vi "Real BC Test.vi"() -> ()   [LabVIEW 2016]
uses:
  Frames & Messages/TypeDefs/Message Config.ctl
  Frames & Messages/TypeDefs/Command Config.ctl
  Frames & Messages/TypeDefs/Message Control.ctl
  1553 SubComponent/TypeDefs/Parameter Table Data.ctl
  1553 SubComponent/TypeDefs/Scaling Information.ctl
  Bus Controller/TypeDefs/Bus Controller Configuration.ctl
  Frames & Messages/TypeDefs/Async Message Config.ctl
  Frames & Messages/TypeDefs/Async RT-RT Message Config.ctl
  1553 Board/1553 Board.lvclass/1553 Board.ctl
  Bus Controller/Bus Controller.lvclass
  D:/SVN/Products/BCI-1553/Software/Development/2016/RealTime/1553 SubComponent/1553 SubComponent.lvclass
  <vilib>/Utility/file.llb/Write Delimited Spreadsheet (string).vi
  1553 Component/1553 Component.lvclass
  Frames & Messages/Major Frame/Major Frame.lvclass
  1553 Board/1553 Board.lvclass
  Utilities/FPGA Interface/FPGA Interface.lvclass
  Frames & Messages/Async Message/Async Message.lvclass
  Frames & Messages/Message/Message.lvclass
  BCI-1553 API.lvlib
  1553 SubComponent/1553 SubComponent.lvclass
  Frames & Messages/Minor Frame/Minor Frame.lvclass
  Frames & Messages/Async RT-RT Message/Async RT-RT Message.lvclass
  D:/SVN/Products/BCI-1553/Software/Development/2016/RealTime/Frames & Messages/Async Message/Async Message.lvclass
panel:
  in  "Async Value":dbl format="%#_13g"
  in  "Async Param":string="Async Param"
  in  "Send Async":bool
  in  "Component ID (1-8)":u8=1
  in  "Update Param":bool
  in  "Scaled Data 2":dbl[](array[numeric])
  in  "Parameters 2":string[](array[string])
  out "Scaled Data":dbl[][](array[numeric])
  out "Parameters":string[][](array[string])
  in  "Holt Memory dump":path
  in  "Holt Memory to File":bool
  in  "Addresses to Read":u16 format="%0.0f"
  out "Data":u16[](array[numeric]) format="%04x"
  in  "Addr":u16 format="%04x"
  in  "Read":bool
  out "error out":errorcluster
  in  "stop":bool
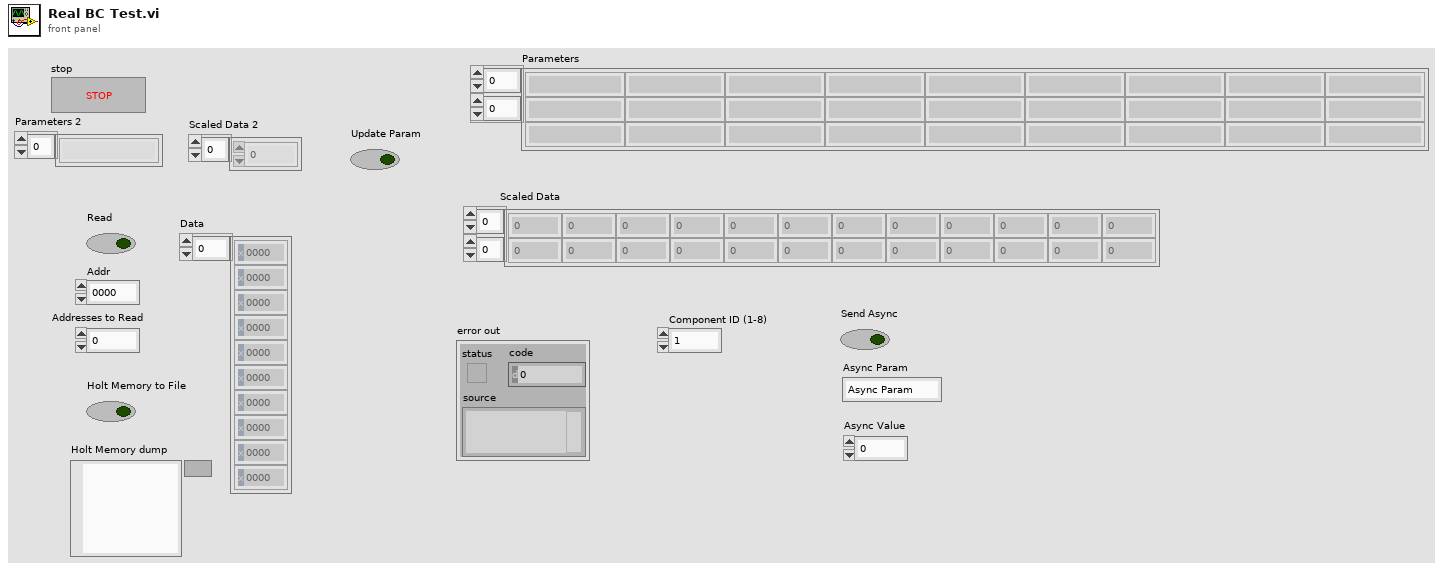
[diagram p1: front panel]
types:
  T1 = typedef "BCI-1553 API.lvlib/Async RT-RT Message Config.ctl" = cluster{"Tx Command Config":T2}
  T2 = typedef "BCI-1553 API.lvlib/Command Config.ctl" = cluster{"Command Type":enum16{"Transmit", "Receive"}, "Terminal Address (0-30)":u16, "SubAddress (1-30)":u16, "WC/MC (1-32)":u16, "Command Data":u16[]}
  T3 = typedef "BCI-1553 API.lvlib/1553 SubComponent.lvclass/Parameter Table Data.ctl" = cluster{"Parameter Name":string, "Base Word":u16, "Address":u16, "Value":u64, "Mask":u16[], "Scaling Info":T4}
  T4 = typedef "BCI-1553 API.lvlib/1553 SubComponent.lvclass/Scaling Information.ctl" = cluster{"Bit Offset":i32, "Bit Count":i32, "LSB Resolution":dbl, "2's Complement":bool, "Big Endian":bool, "Sign Bit":bool}
  T5 = typedef "BCI-1553 API.lvlib/Async Message Config.ctl" = cluster{"Group":i32, "High Priority":bool, "Time to Next Msg (100 us)":u16, "Command Config":T2, "Message Control":T6}
  T6 = typedef "BCI-1553 API.lvlib/Message Control.ctl" = cluster{"MC17 Time Sync":bool, "Error Mask":bool, "Service Request Mask":bool, "Busy Mask":bool, "SubSystem Flag Mask":bool, "Terminal Flag Mask":bool, "Reserved Mask":bool, "Retry":bool, "Bus A / !Bus B":bool, "Self-Test Loopback":bool, "Broadcast Mask":bool, "EoM Interrupt":bool, "Mode Code Format":bool, "Broadcast Format":bool, "RT-RT Format":bool}
  T7 = typedef "BCI-1553 API.lvlib/Message Config.ctl" = cluster{"Time to Next Msg (4 us)":u16, "Command Config":T2, "Message Control":T6}
  T8 = typedef "BCI-1553 API.lvlib/Bus Controller.lvclass/Bus Controller Configuration.ctl" = cluster{"BC Timeout":u16, "BC Retry":bool, "BC Second Retry":bool, "BC Retry Alt Bus":bool, "BC Second Retry Alt Bus":bool, "BC Retry on Status Bit":bool, "Msg Error No Data Valid":bool, "Busy Status No Data Valid":bool, "Msg Gap Timer":bool, "Watchdog Timer":bool, "Time Tag Sync":bool, "Even Time Tag Sync":bool, "Gap Check":bool, "Broadcast Mask Enable":bool}
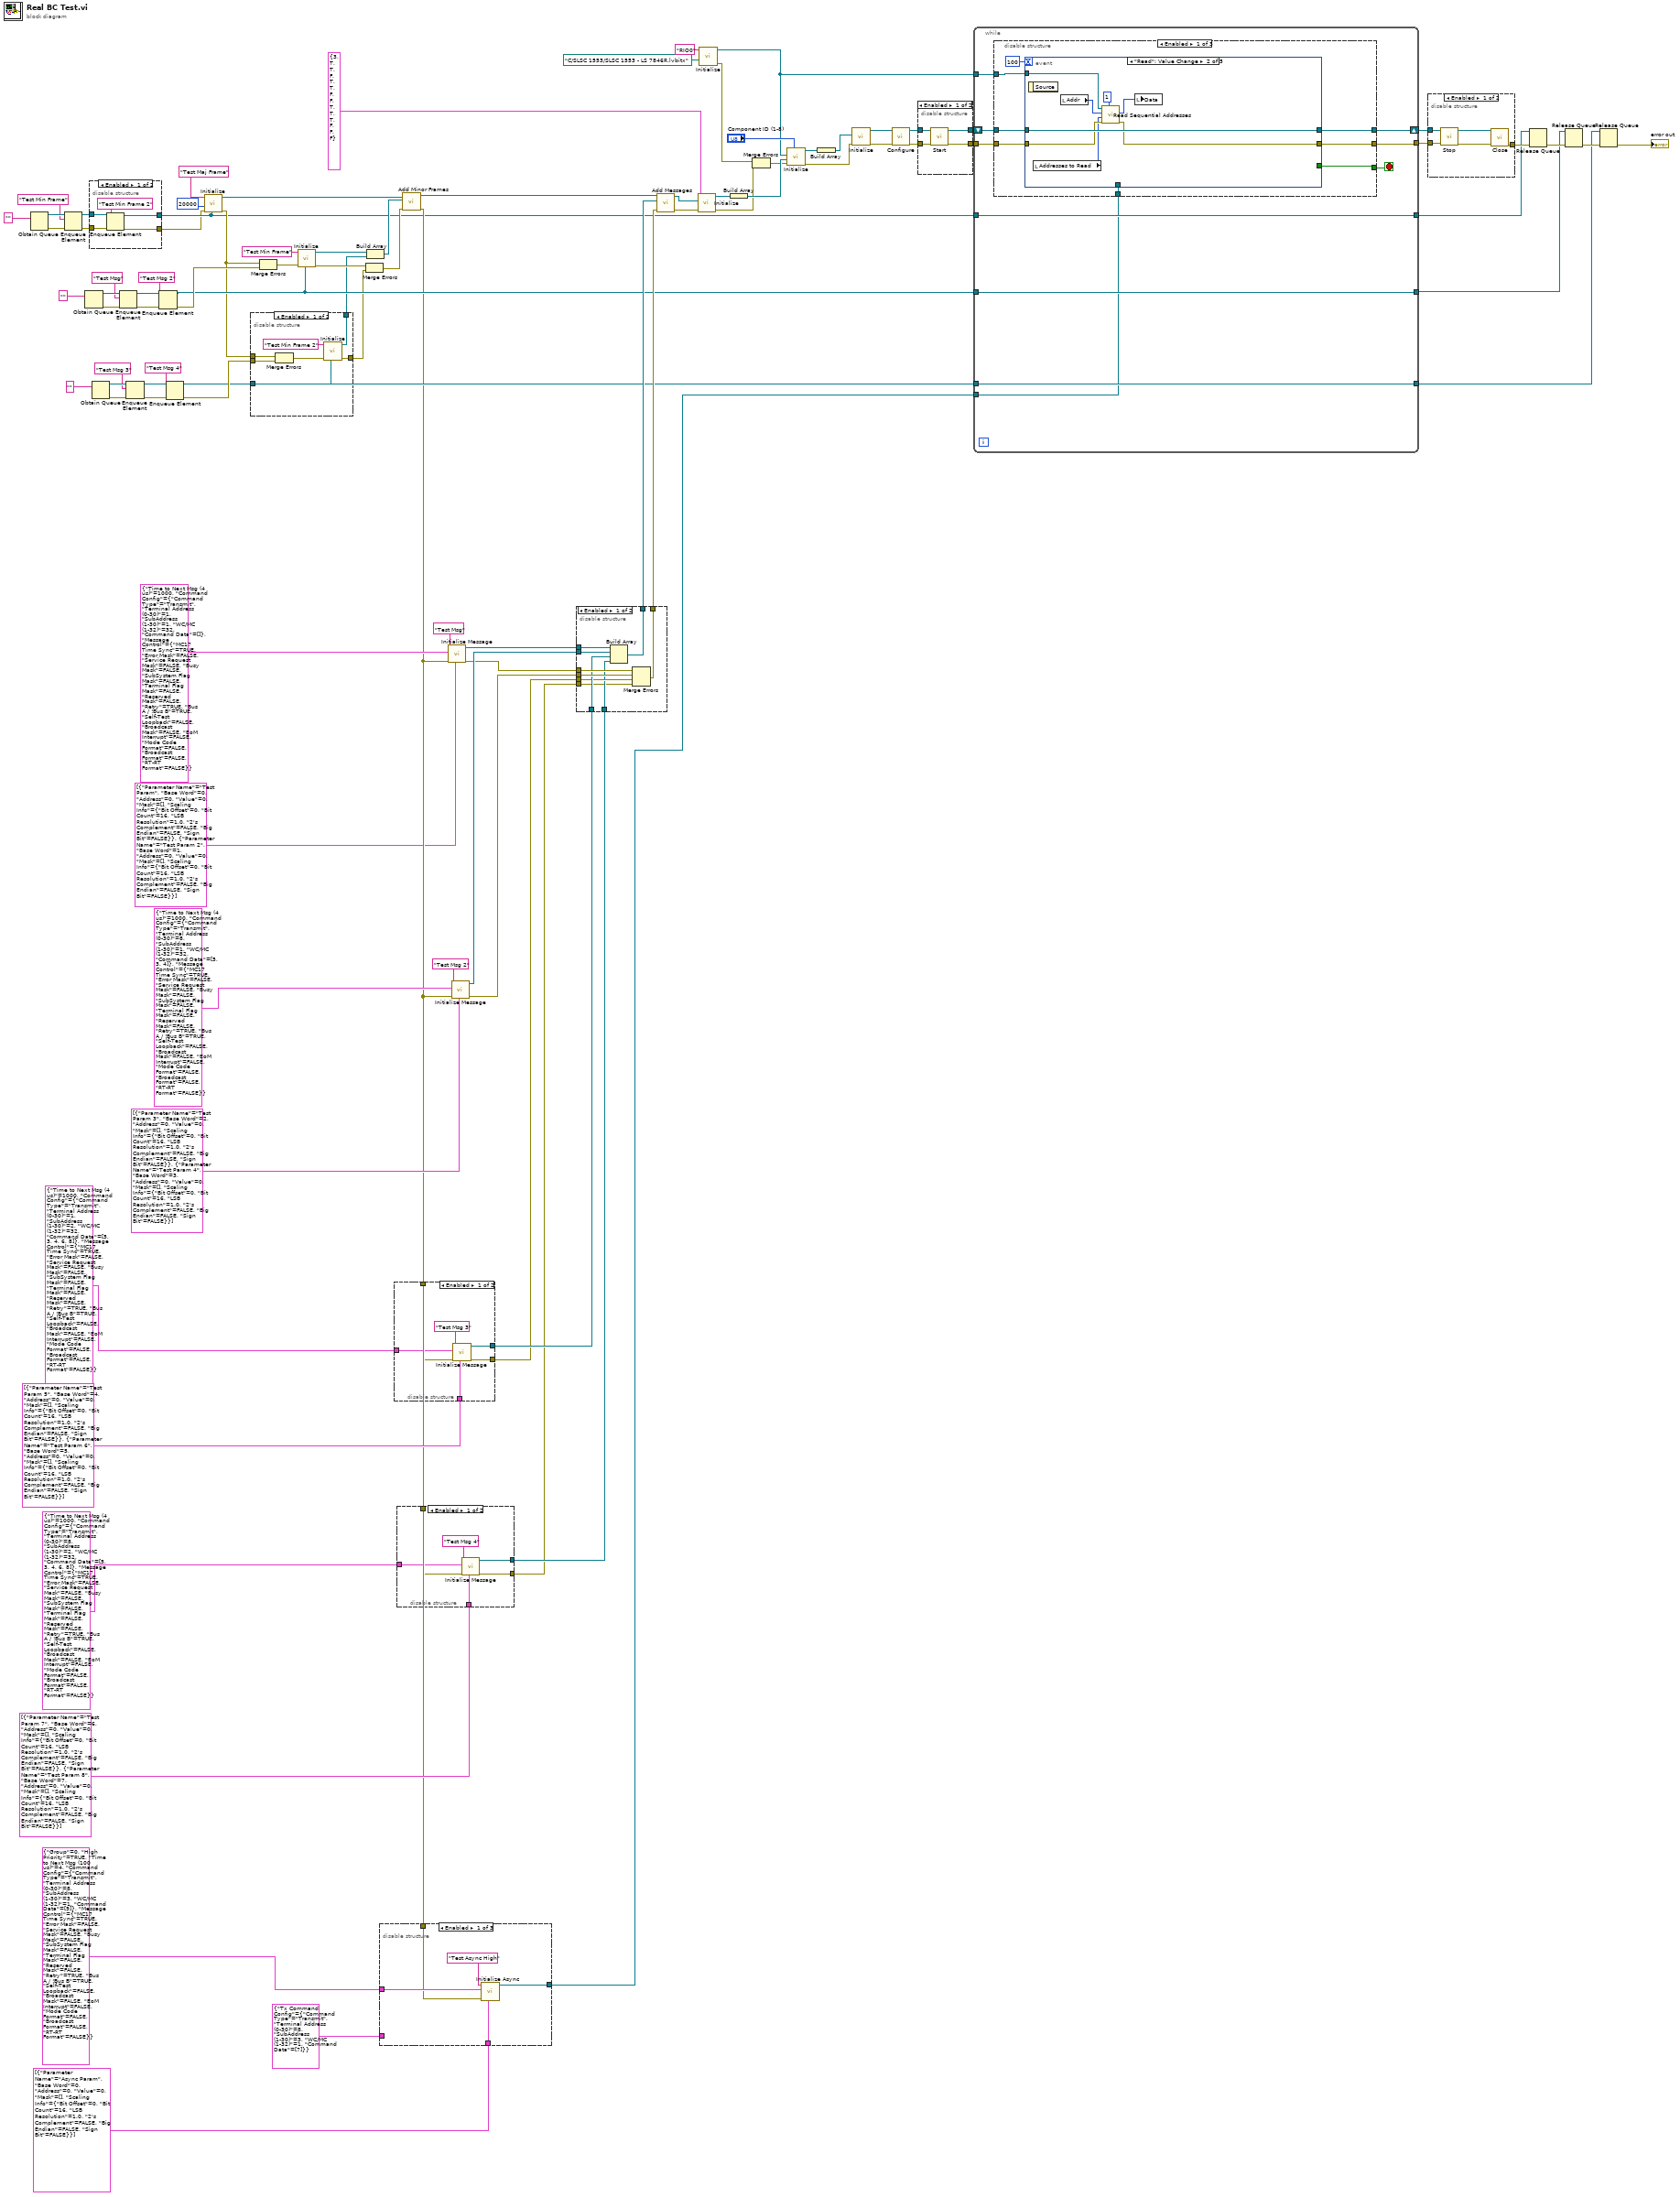
[diagram p0: block diagram]
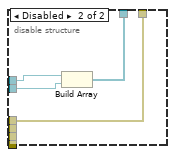
[diagram p4: hidden frame]
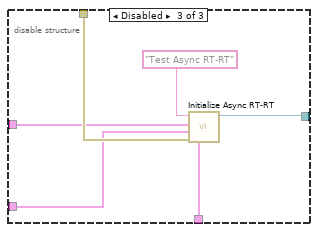
[diagram p8: hidden frame]
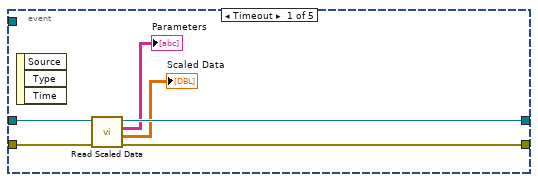
[diagram p11: hidden frame]
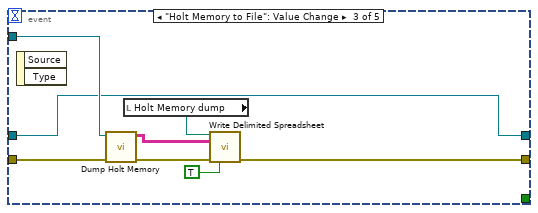
[diagram p12: hidden frame]
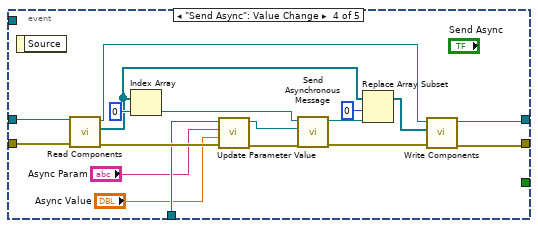
[diagram p13: hidden frame]
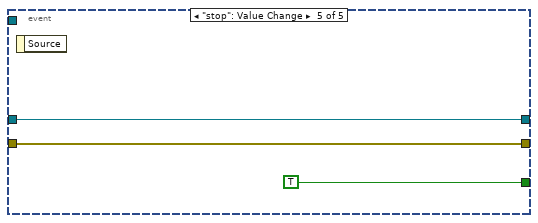
[diagram p14: hidden frame]
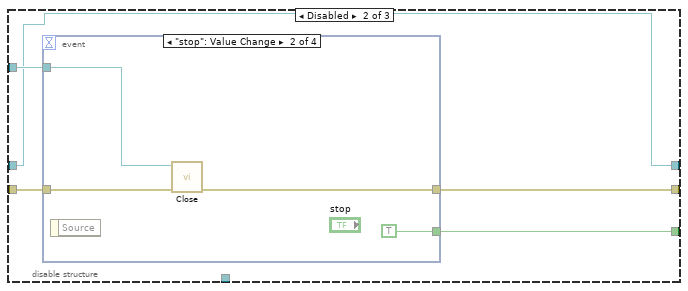
[diagram p15: hidden frame]
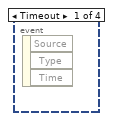
[diagram p16: hidden frame]
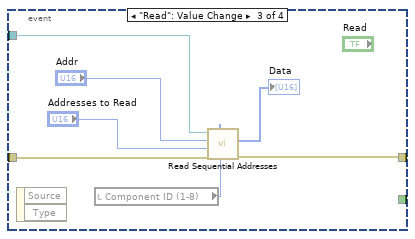
[diagram p17: hidden frame]
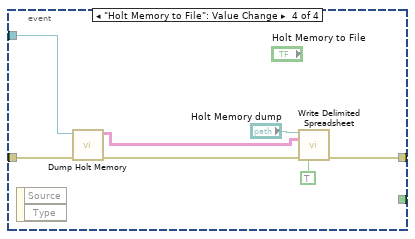
[diagram p18: hidden frame]
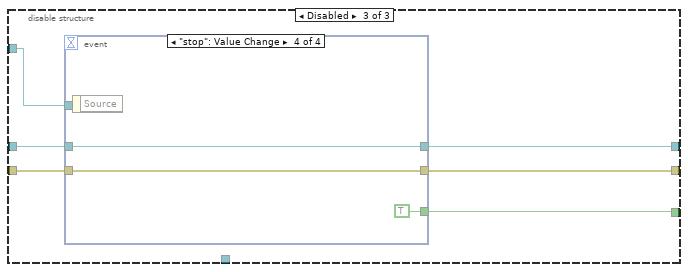
[diagram p19: hidden frame]
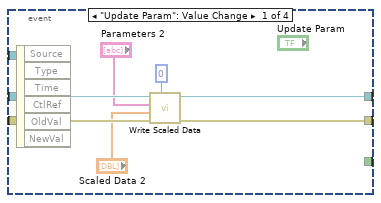
[diagram p20: hidden frame]
diagram:
  n1 = Obtain Queue(element data type="") -> (queue out=w69:refnum<queue>, error out=w70:errorcluster)  [unwired: 4 in, 1 out]
  n2 = Enqueue Element(queue=w69, element="Test Min Frame", error in (no error)=w70) -> (queue out=w10:refnum<queue>, error out=w11:errorcluster)  [unwired: 1 in, 1 out]
  n3 = Obtain Queue(element data type="") -> (queue out=w57:refnum<queue>, error out=w58:errorcluster)  [unwired: 4 in, 1 out]
  n4 = disable-structure shown="Enabled" {
    disable-tunnel: w11 -> [w99 w100]
    disable-tunnel: w10 -> [w98 w101]
    disable-tunnel: [w96 w101] -> w5
    disable-tunnel: [w95 w100] -> w4
    frame Enabled {
      n5 = Enqueue Element(queue=w98, element="Test Min Frame 2", error in (no error)=w99) -> (queue out=w96:refnum<queue>, error out=w95:errorcluster)  [unwired: 1 in, 1 out]
    }
    frame Disabled {
    }
  }
  n6 = Obtain Queue(element data type="") -> (queue out=w34:refnum<queue>, error out=w35:errorcluster)  [unwired: 4 in, 1 out]
  n7 = Enqueue Element(queue=w57, element="Test Msg", error in (no error)=w58) -> (queue out=w39:refnum<queue>, error out=w40:errorcluster)  [unwired: 1 in, 1 out]
  n8 = Enqueue Element(queue=w34, element="Test Msg 3", error in (no error)=w35) -> (queue out=w30:refnum<queue>, error out=w31:errorcluster)  [unwired: 1 in, 1 out]
  n9 = Enqueue Element(queue=w39, element="Test Msg 2", error in (no error)=w40) -> (queue out=w37:refnum<queue>, error out=w38:errorcluster)  [unwired: 1 in, 1 out]
  n10 = Enqueue Element(queue=w30, element="Test Msg 4", error in (no error)=w31) -> (queue out=w22:refnum<queue>, error out=w24:errorcluster)  [unwired: 1 in, 1 out]
  n11 = call "Initialize.vi"("Schedule"=w5, "error in (no error)"=w4, "Minor Frame Time (100 us)"=u16 20000 ("Minor Frame Time (us)"), "ID"="Test Maj Frame") -> ("error out"=w25:errorcluster, "Major Frame out"=w53:refnum<class "Major Frame.lvclass">)  [unwired: 6 in]
  n12 = disable-structure shown="Enabled" {
    disable-tunnel: [w107 w109] -> w27
    disable-tunnel: w25 -> [w106 w109]
    disable-tunnel: w24 -> [w104 _]
    disable-tunnel: w22 -> [w103 _]
    disable-tunnel: [w102 _] -> w1
    frame Enabled {
      n13 = Merge Errors(w106, w104) -> (w105:errorcluster)
      n14 = call "Initialize.vi"("Schedule"=w103, "error in (no error)"=w105, "ID"="Test Min Frame 2") -> ("error out"=w107:errorcluster, "Minor Frame out"=w102:refnum<class "Minor Frame.lvclass">)  [unwired: 7 in]
    }
    frame Disabled {
    }
  }
  n15 = Merge Errors(w25, w38) -> (w54:errorcluster)
  n16 = call "Initialize.vi"("Schedule"=w37, "error in (no error)"=w54, "ID"="Test Min Frame") -> ("error out"=w28:errorcluster, "Minor Frame out"=w52:refnum<class "Minor Frame.lvclass">)  [unwired: 7 in]
  n17 = Merge Errors(w28, w27) -> (w26:errorcluster)
  n18 = Build Array(w52, w1) -> (w51:refnum<class "Minor Frame.lvclass">[])
  n19 = call-dynamic "Add Minor Frames.vi"("error in (no error)"=w26, "Minor Frames"=w51, "Major Frame in"=w53) -> ("error out"=w7:errorcluster, "Major Frame out"=w50:refnum<class "Major Frame.lvclass">)  [unwired: 7 in]
  n20 = disable-structure shown="Enabled" {
    disable-tunnel: T5 {"Group"=0, "High Priority"=TRUE, "Time to Next Msg (100 us)"=4, "Command Config"={"Command Type"=enum."Transmit", "Terminal Address (0-30)"=8, "SubAddress (1-30)"=3, "WC/MC (1-32)"=1, "Command Data"=[9]}, "Message Control"={"MC17 Time Sync"=TRUE, "Error Mask"=FALSE, "Service Request Mask"=FALSE, "Busy Mask"=FALSE, "SubSystem Flag Mask"=FALSE, "Terminal Flag Mask"=FALSE, "Reserved Mask"=FALSE, "Retry"=TRUE, "Bus A / !Bus B"=TRUE, "Self-Test Loopback"=FALSE, "Broadcast Mask"=FALSE, "EoM Interrupt"=FALSE, "Mode Code Format"=FALSE, "Broadcast Format"=FALSE, "RT-RT Format"=FALSE}} ("Async Message Config") -> [w113 _ w116]
    disable-tunnel: T3[] [{"Parameter Name"="Async Param", "Base Word"=0, "Address"=0, "Value"=0, "Mask"=[], "Scaling Info"={"Bit Offset"=0, "Bit Count"=16, "LSB Resolution"=1.0, "2's Complement"=FALSE, "Big Endian"=FALSE, "Sign Bit"=FALSE}}] ("Parameters") -> [w112 _ w120]
    disable-tunnel: w7 -> [w111 _ w118]
    disable-tunnel: [w110 _ w119] -> w6
    disable-tunnel: T1 {"Tx Command Config"={"Command Type"=enum."Transmit", "Terminal Address (0-30)"=8, "SubAddress (1-30)"=3, "WC/MC (1-32)"=1, "Command Data"=[7]}} ("RT-RT Async Message Config") -> [_ _ w117]
    frame Enabled {
      n21 = call "Initialize Async.vi"("Parameters"=w112, "error in (no error)"=w111, "Async Message Config"=w113, "ID"="Test Async High") -> ("Async Message out"=w110:refnum<class "Async Message.lvclass">)  [unwired: 6 in, 1 out]
    }
    frame Disabled {
    }
    frame Disabled {
      n22 = call "Initialize Async RT-RT.vi"("Parameters"=w120, "error in (no error)"=w118, "RT-RT Async Message Config"=w117, "Async Message Config"=w116, "ID"="Test Async RT-RT") -> ("Async RT-RT Message out"=w119:refnum<class "Async RT-RT Message.lvclass">)  [unwired: 5 in, 1 out]
    }
  }
  n23 = disable-structure shown="Enabled" {
    disable-tunnel: [w125 _] -> w19
    disable-tunnel: [w124 _] -> w18
    disable-tunnel: T7 {"Time to Next Msg (4 us)"=1000, "Command Config"={"Command Type"=enum."Transmit", "Terminal Address (0-30)"=1, "SubAddress (1-30)"=2, "WC/MC (1-32)"=32, "Command Data"=[5, 3, 4, 6, 8]}, "Message Control"={"MC17 Time Sync"=TRUE, "Error Mask"=FALSE, "Service Request Mask"=FALSE, "Busy Mask"=FALSE, "SubSystem Flag Mask"=FALSE, "Terminal Flag Mask"=FALSE, "Reserved Mask"=FALSE, "Retry"=TRUE, "Bus A / !Bus B"=TRUE, "Self-Test Loopback"=FALSE, "Broadcast Mask"=FALSE, "EoM Interrupt"=FALSE, "Mode Code Format"=FALSE, "Broadcast Format"=FALSE, "RT-RT Format"=FALSE}} ("Message  Config") -> [w123 _]
    disable-tunnel: T3[] [{"Parameter Name"="Test Param 5", "Base Word"=4, "Address"=0, "Value"=0, "Mask"=[], "Scaling Info"={"Bit Offset"=0, "Bit Count"=16, "LSB Resolution"=1.0, "2's Complement"=FALSE, "Big Endian"=FALSE, "Sign Bit"=FALSE}}, {"Parameter Name"="Test Param 6", "Base Word"=5, "Address"=0, "Value"=0, "Mask"=[], "Scaling Info"={"Bit Offset"=0, "Bit Count"=16, "LSB Resolution"=1.0, "2's Complement"=FALSE, "Big Endian"=FALSE, "Sign Bit"=FALSE}}] ("Parameters") -> [w122 _]
    disable-tunnel: w7 -> [w121 _]
    frame Enabled {
      n24 = call "Initialize Message.vi"("Parameters"=w122, "error in (no error)"=w121, "Message  Config"=w123, "ID"="Test Msg 3") -> ("error out"=w124:errorcluster, "Message out"=w125:refnum<class "Message.lvclass">)  [unwired: 6 in]
    }
    frame Disabled {
    }
  }
  n25 = disable-structure shown="Enabled" {
    disable-tunnel: [w131 _] -> w17
    disable-tunnel: [w130 _] -> w16
    disable-tunnel: T7 {"Time to Next Msg (4 us)"=1000, "Command Config"={"Command Type"=enum."Transmit", "Terminal Address (0-30)"=8, "SubAddress (1-30)"=2, "WC/MC (1-32)"=32, "Command Data"=[5, 3, 4, 6, 8]}, "Message Control"={"MC17 Time Sync"=TRUE, "Error Mask"=FALSE, "Service Request Mask"=FALSE, "Busy Mask"=FALSE, "SubSystem Flag Mask"=FALSE, "Terminal Flag Mask"=FALSE, "Reserved Mask"=FALSE, "Retry"=TRUE, "Bus A / !Bus B"=TRUE, "Self-Test Loopback"=FALSE, "Broadcast Mask"=FALSE, "EoM Interrupt"=FALSE, "Mode Code Format"=FALSE, "Broadcast Format"=FALSE, "RT-RT Format"=FALSE}} ("Message  Config") -> [w129 _]
    disable-tunnel: T3[] [{"Parameter Name"="Test Param 7", "Base Word"=6, "Address"=0, "Value"=0, "Mask"=[], "Scaling Info"={"Bit Offset"=0, "Bit Count"=16, "LSB Resolution"=1.0, "2's Complement"=FALSE, "Big Endian"=FALSE, "Sign Bit"=FALSE}}, {"Parameter Name"="Test Param 8", "Base Word"=7, "Address"=0, "Value"=0, "Mask"=[], "Scaling Info"={"Bit Offset"=0, "Bit Count"=16, "LSB Resolution"=1.0, "2's Complement"=FALSE, "Big Endian"=FALSE, "Sign Bit"=FALSE}}] ("Parameters") -> [w128 _]
    disable-tunnel: w7 -> [w127 _]
    frame Enabled {
      n26 = call "Initialize Message.vi"("Parameters"=w128, "error in (no error)"=w127, "Message  Config"=w129, "ID"="Test Msg 4") -> ("error out"=w130:errorcluster, "Message out"=w131:refnum<class "Message.lvclass">)  [unwired: 6 in]
    }
    frame Disabled {
    }
  }
  n27 = call "Initialize Message.vi"("Parameters"=T3[] [{"Parameter Name"="Test Param", "Base Word"=0, "Address"=0, "Value"=0, "Mask"=[], "Scaling Info"={"Bit Offset"=0, "Bit Count"=16, "LSB Resolution"=1.0, "2's Complement"=FALSE, "Big Endian"=FALSE, "Sign Bit"=FALSE}}, {"Parameter Name"="Test Param 2", "Base Word"=1, "Address"=0, "Value"=0, "Mask"=[], "Scaling Info"={"Bit Offset"=0, "Bit Count"=16, "LSB Resolution"=1.0, "2's Complement"=FALSE, "Big Endian"=FALSE, "Sign Bit"=FALSE}}], "error in (no error)"=w7, "Message  Config"=T7 {"Time to Next Msg (4 us)"=1000, "Command Config"={"Command Type"=enum."Transmit", "Terminal Address (0-30)"=1, "SubAddress (1-30)"=1, "WC/MC (1-32)"=32, "Command Data"=[]}, "Message Control"={"MC17 Time Sync"=TRUE, "Error Mask"=FALSE, "Service Request Mask"=FALSE, "Busy Mask"=FALSE, "SubSystem Flag Mask"=FALSE, "Terminal Flag Mask"=FALSE, "Reserved Mask"=FALSE, "Retry"=TRUE, "Bus A / !Bus B"=TRUE, "Self-Test Loopback"=FALSE, "Broadcast Mask"=FALSE, "EoM Interrupt"=FALSE, "Mode Code Format"=FALSE, "Broadcast Format"=FALSE, "RT-RT Format"=FALSE}}, "ID"="Test Msg") -> ("error out"=w45:errorcluster, "Message out"=w92:refnum<class "Message.lvclass">)  [unwired: 6 in]
  n28 = call "Initialize Message.vi"("Parameters"=T3[] [{"Parameter Name"="Test Param 3", "Base Word"=2, "Address"=0, "Value"=0, "Mask"=[], "Scaling Info"={"Bit Offset"=0, "Bit Count"=16, "LSB Resolution"=1.0, "2's Complement"=FALSE, "Big Endian"=FALSE, "Sign Bit"=FALSE}}, {"Parameter Name"="Test Param 4", "Base Word"=3, "Address"=0, "Value"=0, "Mask"=[], "Scaling Info"={"Bit Offset"=0, "Bit Count"=16, "LSB Resolution"=1.0, "2's Complement"=FALSE, "Big Endian"=FALSE, "Sign Bit"=FALSE}}], "error in (no error)"=w7, "Message  Config"=T7 {"Time to Next Msg (4 us)"=1000, "Command Config"={"Command Type"=enum."Transmit", "Terminal Address (0-30)"=8, "SubAddress (1-30)"=1, "WC/MC (1-32)"=32, "Command Data"=[5, 3, 4]}, "Message Control"={"MC17 Time Sync"=TRUE, "Error Mask"=FALSE, "Service Request Mask"=FALSE, "Busy Mask"=FALSE, "SubSystem Flag Mask"=FALSE, "Terminal Flag Mask"=FALSE, "Reserved Mask"=FALSE, "Retry"=TRUE, "Bus A / !Bus B"=TRUE, "Self-Test Loopback"=FALSE, "Broadcast Mask"=FALSE, "EoM Interrupt"=FALSE, "Mode Code Format"=FALSE, "Broadcast Format"=FALSE, "RT-RT Format"=FALSE}}, "ID"="Test Msg 2") -> ("error out"=w43:errorcluster, "Message out"=w46:refnum<class "Message.lvclass">)  [unwired: 6 in]
  n29 = disable-structure shown="Enabled" {
    disable-tunnel: w92 -> [w142 w146]
    disable-tunnel: [w141 w144] -> w91
    disable-tunnel: w46 -> [w140 w145]
    disable-tunnel: w45 -> [w139 w143]
    disable-tunnel: [w138 w143] -> w44
    disable-tunnel: w43 -> [w137 _]
    disable-tunnel: w19 -> [w136 _]
    disable-tunnel: w18 -> [w135 _]
    disable-tunnel: w17 -> [w134 _]
    disable-tunnel: w16 -> [w133 _]
    frame Enabled {
      n30 = Build Array(w142, w140, w136, w134) -> (w141:refnum<class "Message.lvclass">[])
      n31 = Merge Errors(w139, w137, w135, w133) -> (w138:errorcluster)
    }
    frame Disabled {
      n32 = Build Array(w146, w145) -> (w144:refnum<class "Message.lvclass">[])
    }
  }
  n33 = call-dynamic "Add Messages.vi"("error in (no error)"=w44, "Messages"=w91, "Major Frame in"=w50) -> ("error out"=w90:errorcluster, "Major Frame out"=w89:refnum<class "Major Frame.lvclass">)  [unwired: 7 in]
  n34 = call "Initialize.vi"("error in (no error)"=w90, "Major Frame"=w89, "Configuration"=T8 {"BC Timeout"=3, "BC Retry"=TRUE, "BC Second Retry"=TRUE, "BC Retry Alt Bus"=FALSE, "BC Second Retry Alt Bus"=TRUE, "BC Retry on Status Bit"=TRUE, "Msg Error No Data Valid"=FALSE, "Busy Status No Data Valid"=FALSE, "Msg Gap Timer"=TRUE, "Watchdog Timer"=TRUE, "Time Tag Sync"=TRUE, "Even Time Tag Sync"=FALSE, "Gap Check"=FALSE, "Broadcast Mask Enable"=FALSE}) -> ("error out"=w64:errorcluster, "Bus Controller out"=w87:refnum<class "Bus Controller.lvclass">)  [unwired: 7 in]
  n35 = call "Initialize.vi"("Bitfile path"=path "C:/SLSC 1553/SLSC 1553 - LS 7846R.lvbitx", "Device address"="RIO0") -> ("error out"=w63:errorcluster, "FPGA Interface out"=w60:refnum<class "FPGA Interface.lvclass">)  [unwired: 8 in]
  n36 = Build Array(w87) -> (w86:refnum<class "Bus Controller.lvclass">[])
  n37 = Merge Errors(w63, w64) -> (w62:errorcluster)
  n38 = call "Initialize.vi"("Component ID (1-8)"="Component ID (1-8)", "error in (no error)"=w62, "SubComponents"=w86, "FPGA Interface"=w60) -> ("error out"=w83:errorcluster, "1553 Component out"=w85:refnum<class "1553 Component.lvclass">)  [unwired: 6 in]
  n39 = Build Array(w85) -> (w84:refnum<class "1553 Component.lvclass">[])
  n40 = call "Initialize.vi"("error in (no error)"=w83, "Components"=w84) -> ("error out"=w82:errorcluster, "1553 Board out"=w81:refnum<class "1553 Board.lvclass">)  [unwired: 8 in]
  n41 = call-dynamic "Configure.vi"("error in (no error)"=w82, "1553 Board in"=w81) -> ("error out"=w80:errorcluster, "1553 Board out"=w79:refnum<class "1553 Board.lvclass">)  [unwired: 8 in]
  n42 = disable-structure shown="Enabled" {
    disable-tunnel: w80 -> [w150 w151]
    disable-tunnel: w79 -> [w149 w152]
    disable-tunnel: [w148 w151] -> w78
    disable-tunnel: [w147 w152] -> w77
    frame Enabled {
      n43 = call-dynamic "Start.vi"("error in (no error)"=w150, "1553 Board in"=w149) -> ("error out"=w148:errorcluster, "1553 Board out"=w147:refnum<class "1553 Board.lvclass">)  [unwired: 8 in]
    }
    frame Disabled {
    }
  }
  n44 = while {
    tunnel: w78 -> [w160]
    tunnel: [w159] -> w76
    tunnel: w5 -> [w162]
    tunnel: [w162] -> w65
    tunnel: w60 -> [w158]
    tunnel: w37 -> [w155]
    tunnel: [w155] -> w48
    tunnel: w22 -> [w154]
    tunnel: [w154] -> w21
    tunnel: w6 -> [w153]
    shift-right: [w156] -> w75
    shift-left: w77 -> [w157]
    stop <- w161 stop-if-true
    n45 = disable-structure shown="Enabled" {
      disable-tunnel: [w165 w218 w238] -> w161
      disable-tunnel: w160 -> [w170 w217 w242]
      disable-tunnel: [w168 w216 w240] -> w159
      disable-tunnel: w158 -> [w166 w215 w237]
      disable-tunnel: w157 -> [w169 w214 w241]
      disable-tunnel: [w167 w214 w239] -> w156
      disable-tunnel: w153 -> [w163 _ _]
      frame Enabled {
        n46 = event shown="[1] \"Read\": Value Change" {
          selector: _ -> [_ _ _ _ _]
          dyn-events: _ -> [_ _ _ _ _]
          timeout: 100 -> [_ _ _ _ _]
          tunnel: w170 -> [w176 w183 w192 w210 w212]
          tunnel: w169 -> [w175 w184 w186 w209 w213]
          tunnel: [w174 w182 w187 w199 w212] -> w168
          tunnel: [w173 w184 w186 w198 w213] -> w167
          tunnel: w166 -> [_ w181 w191 _ _]
          tunnel: [_ _ _ _ TRUE] -> w165
          tunnel: w163 -> [_ _ _ w205 _]
          event Timeout {
            n47 = event-data() -> ()  [unwired: 1 in, 3 out]
            n48 = call-dynamic "Read Scaled Data.vi"("error in (no error)"=w176, "1553 Board in"=w175) -> ("error out"=w174:errorcluster, "Scaled Data"=→"Scaled Data":dbl[][], "Parameters"=→"Parameters":string[][], "1553 Board out"=w173:refnum<class "1553 Board.lvclass">)  [unwired: 6 in]
          }
          event "Read": Value Change {
            n49 = event-data() -> ()  [unwired: 1 in, 1 out]
            n50 = local read "Addresses to Read"() -> (w178:u16)
            n51 = local read "Addr"() -> (w179:u16)
            n52 = call-dynamic "Read Sequential Addresses.vi"("Target IC (1-8)"=u8 1, "error in (no error)"=w183, "Addresses to Read"=w178, "Starting Address"=w179, "FPGA Interface in"=w181) -> ("error out"=w182:errorcluster, "Data"=w177:u16[])  [unwired: 5 in]
            n53 = local write "Data"(w177) -> ()
          }
          event "Holt Memory to File": Value Change {
            n54 = event-data() -> ()  [unwired: 1 in, 2 out]
            n55 = call "Dump Holt Memory.vi"("error IO"=w192, "FPGA Interface"=w191) -> ("error out"=w190:errorcluster, "appended array"=w189:string[][])  [unwired: 8 in]
            n56 = local read "Holt Memory dump"() -> (w185:path)
            n57 = call-poly <vilib>:"Write Delimited Spreadsheet.vi"("file path (dialog if empty)"=w185, "2D data"=w189, "error in (no error)"=w190, "transpose? (no:F)"=TRUE) -> ("error out"=w187:errorcluster)  [unwired: 10 in, 1 out]
          }
          event "Send Async": Value Change {
            n58 = event-data() -> ()  [unwired: 1 in, 1 out]
            n59 = call "Read Components.vi"("error in (no error)"=w210, "1553 Board in"=w209) -> ("error out"=w207:errorcluster, "Components"=w196:refnum<class "1553 Component.lvclass">[], "1553 Board out"=w197:refnum<class "1553 Board.lvclass">)  [unwired: 7 in]
            n60 = Index Array(array=w196, index=0) -> (element=w203:refnum<class "1553 Component.lvclass">)
            n61 = call-dynamic "Update Parameter Value.vi"("error in (no error)"=w207, "Value"="Async Value", "Parameter"="Async Param", "Async Message in"=w205) -> ("error out"=w206:errorcluster, "Async Message out"=w204:refnum<class "Async Message.lvclass">)  [unwired: 6 in]
            n62 = call-dynamic "Send Asynchronous Message.vi"("error in (no error)"=w206, "Async Message"=w204, "1553 Component in"=w203) -> ("error out"=w200:errorcluster, "1553 Component out"=w195:refnum<class "1553 Component.lvclass">)  [unwired: 7 in]
            n63 = Replace Array Subset(array=w196, new element=w195, index=0) -> (w193:refnum<class "1553 Component.lvclass">[])
            n64 = call "Write Components.vi"("error in (no error)"=w200, "Components"=w193, "1553 Board in"=w197) -> ("error out"=w199:errorcluster, "1553 Board out"=w198:refnum<class "1553 Board.lvclass">)  [unwired: 7 in]
          }
          event "stop": Value Change {
            n65 = event-data() -> ()  [unwired: 1 in, 1 out]
          }
        }
      }
      frame Disabled {
        n66 = event shown="[1] \"stop\": Value Change" {
          selector: _ -> [_ _ _ _]
          dyn-events: _ -> [_ _ _ _]
          timeout: _ -> [_ _ _ _]
          tunnel: [_ TRUE _ _] -> w218
          tunnel: w217 -> [_ w221 w229 w233]
          tunnel: [_ w220 w224 w235] -> w216
          tunnel: w215 -> [_ w219 w228 w232]
          event Timeout {
            n67 = event-data() -> ()  [unwired: 1 in, 3 out]
          }
          event "stop": Value Change {
            n68 = event-data() -> ()  [unwired: 1 in, 1 out]
            n69 = call "Close.vi"("error in (no error)"=w221, "FPGA Interface in"=w219) -> ("error out"=w220:errorcluster)  [unwired: 9 in]
          }
          event "Read": Value Change {
            n70 = event-data() -> ()  [unwired: 1 in, 2 out]
            n71 = local read "Component ID (1-8)"() -> (w223:u8)
            n72 = call-dynamic "Read Sequential Addresses.vi"("Target IC (1-8)"=w223, "error in (no error)"=w229, "Addresses to Read"="Addresses to Read", "Starting Address"="Addr", "FPGA Interface in"=w228) -> ("error out"=w224:errorcluster, "Data"=→"Data":u16[])  [unwired: 5 in]
          }
          event "Holt Memory to File": Value Change {
            n73 = event-data() -> ()  [unwired: 1 in, 2 out]
            n74 = call "Dump Holt Memory.vi"("error IO"=w233, "FPGA Interface"=w232) -> ("error out"=w231:errorcluster, "appended array"=w230:string[][])  [unwired: 8 in]
            n75 = call-poly <vilib>:"Write Delimited Spreadsheet.vi"("file path (dialog if empty)"="Holt Memory dump", "2D data"=w230, "error in (no error)"=w231, "transpose? (no:F)"=TRUE) -> ("error out"=w235:errorcluster)  [unwired: 10 in, 1 out]
          }
        }
      }
      frame Disabled {
        n76 = event shown="[3] \"stop\": Value Change" {
          selector: _ -> [_ _ _ _]
          dyn-events: _ -> [_ _ _ _]
          timeout: _ -> [_ _ _ _]
          tunnel: w242 -> [w249 w255 w264 w267]
          tunnel: w241 -> [w248 w257 w265 w268]
          tunnel: [w244 w250 w263 w267] -> w240
          tunnel: [w243 w257 w265 w268] -> w239
          tunnel: [_ _ _ TRUE] -> w238
          tunnel: w237 -> [_ w256 w262 _]
          event "Update Param": Value Change {
            n77 = event-data() -> ()  [unwired: 1 in, 6 out]
            n78 = call-dynamic "Write Scaled Data.vi"("Component Index"=0, "error in (no error)"=w249, "Scaled Data"="Scaled Data 2", "Parameters"="Parameters 2", "1553 Board in"=w248) -> ("error out"=w244:errorcluster, "1553 Board out"=w243:refnum<class "1553 Board.lvclass">)  [unwired: 5 in]
          }
          event "Holt Memory to File": Value Change {
            n79 = event-data() -> ()  [unwired: 1 in, 1 out]
            n80 = call "Dump Holt Memory.vi"("error IO"=w255, "FPGA Interface"=w256) -> ("error out"=w254:errorcluster, "appended array"=w253:string[][])  [unwired: 8 in]
            n81 = local read "Holt Memory dump"() -> (w251:path)
            n82 = call-poly <vilib>:"Write Delimited Spreadsheet.vi"("file path (dialog if empty)"=w251, "2D data"=w253, "error in (no error)"=w254, "transpose? (no:F)"=TRUE) -> ("error out"=w250:errorcluster)  [unwired: 10 in, 1 out]
          }
          event "Read": Value Change {
            n83 = event-data() -> ()  [unwired: 1 in, 1 out]
            n84 = local read "Addresses to Read"() -> (w259:u16)
            n85 = local read "Addr"() -> (w260:u16)
            n86 = call-dynamic "Read Sequential Addresses.vi"("Target IC (1-8)"=u8 1, "error in (no error)"=w264, "Addresses to Read"=w259, "Starting Address"=w260, "FPGA Interface in"=w262) -> ("error out"=w263:errorcluster, "Data"=w258:u16[])  [unwired: 5 in]
            n87 = local write "Data"(w258) -> ()
          }
          event "stop": Value Change {
            n88 = event-data() -> ()  [unwired: 1 in, 1 out]
          }
        }
      }
    }
  }
  n89 = disable-structure shown="Enabled" {
    disable-tunnel: w76 -> [w273 w274]
    disable-tunnel: w75 -> [w272 _]
    disable-tunnel: [w269 w274] -> w66
    frame Enabled {
      n90 = call-dynamic "Stop.vi"("error in (no error)"=w273, "1553 Board in"=w272) -> ("error out"=w271:errorcluster, "1553 Board out"=w270:refnum<class "1553 Board.lvclass">)  [unwired: 8 in]
      n91 = call-dynamic "Close.vi"("error in (no error)"=w271, "1553 Board in"=w270) -> ("error out"=w269:errorcluster)  [unwired: 9 in]
    }
    frame Disabled {
    }
  }
  n92 = Release Queue(queue=w65, error in (no error)=w66) -> (error out=w49:errorcluster)  [unwired: 1 in, 2 out]
  n93 = Release Queue(queue=w48, error in (no error)=w49) -> (error out=w23:errorcluster)  [unwired: 1 in, 2 out]
  n94 = Release Queue(queue=w21, error in (no error)=w23) -> (error out=→"error out":errorcluster)  [unwired: 1 in, 2 out]
